vi "DAQ AO one shot ch 1.vi"(0 "device name":tag="Dev1", 1 "timeout (s)":dbl=1.0 format="%0.2f", 2 "stop (T)":bool=TRUE, 7 "Heater Voltage":dbl, 11 "error in":errorcluster, 12 "physical channel":string[](array[string])=["ao1"], 13 "channel name":string[](array[string])=["Heater"]) -> (4 "device name out":tag="Dev1", 15 "error out":errorcluster)   [LabVIEW 2019]
doc: "DAQmx NI ELVIS \nAsynchronous AO one shot \nchannel 1\nbug heater\n\nbuilt using the DAQmx assistant\n\nPaul K Dixon\nP3600\nCSUSB Physics\n\nCreates, edits, and runs tasks using NI-DAQmx. Refer to the NI-DAQmx Readme for a complete listing of devices NI-DAQmx supports.\n\nWhen you place this Express VI on the block diagram, the DAQ Assistant launches to create a new task. After you create a task, you can double-click the DAQ Assistant Express VI to edit that task. For continuous measurement or generation, place a while loop around the DAQ Assistant Express VI."
uses:
  <vilib>/DAQmx/write.llb/DAQmx Write.vi
  <vilib>/DAQmx/write.llb/DAQmx Write (Analog 1D DBL NChan 1Samp).vi
  <vilib>/DAQmx/create/channels.llb/DAQmx Create Channel (AO-Voltage-Basic).vi
  <vilib>/DAQmx/miscellaneous.llb/DAQmx Fill In Error Info.vi
panel:
  # "DAQmx NI ELVIS \nAsynchronous AO one shot \nchannel 1\nbug heater"
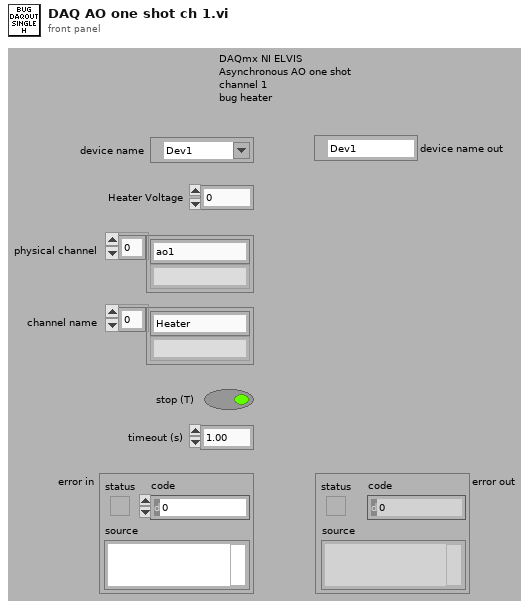
[diagram p1: front panel]
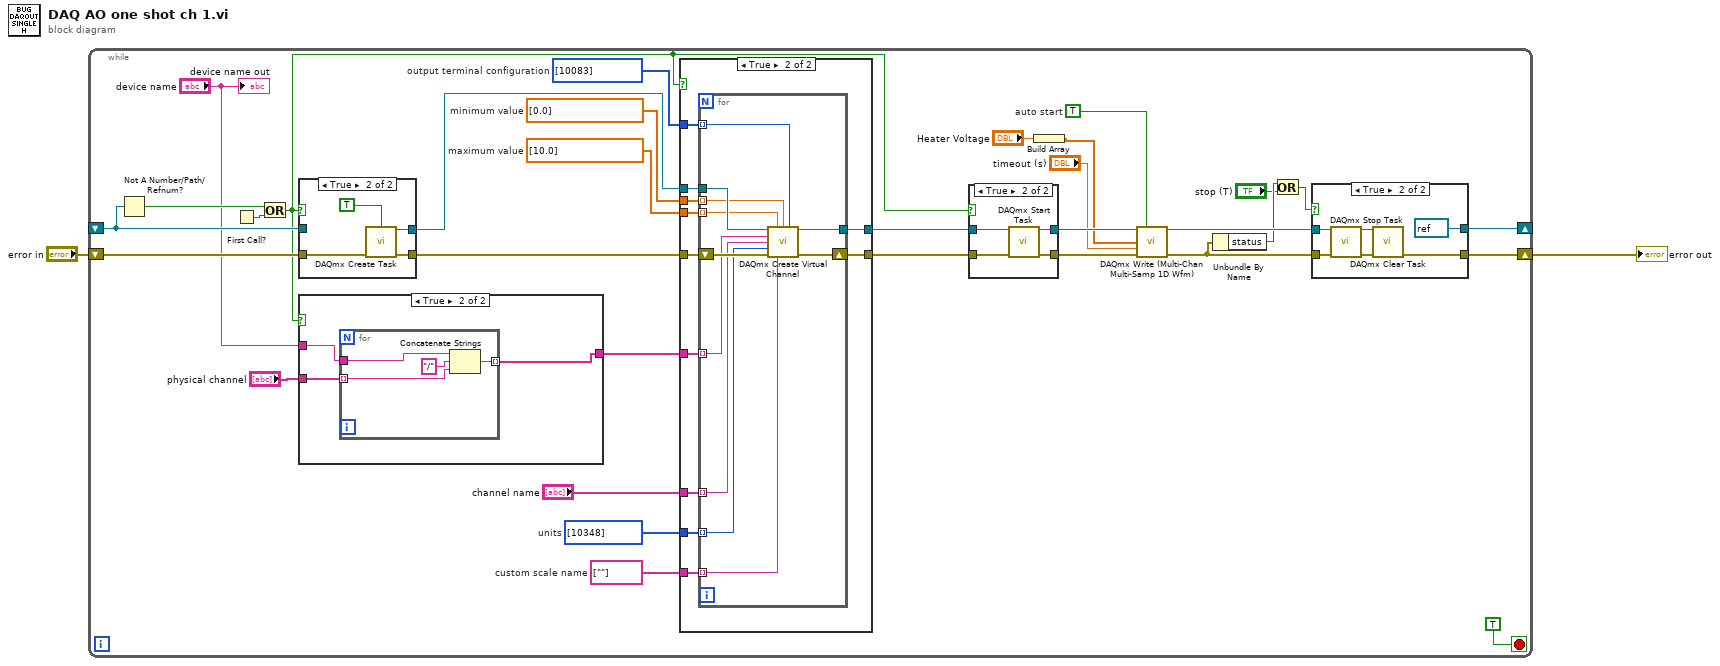
[diagram p0: block diagram]
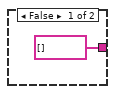
[diagram p5: hidden frame]
diagram:
  n1 = while {
    shift-right: [w11] -> _
    shift-left: _ -> [w31]
    shift-right: [w9] -> w1
    shift-left: "error in" -> [w32]
    stop <- TRUE stop-if-true
    w13 = TRUE  # auto start
    w19 = i32[] [10083] items=["Default"=-1, "RSE"=10083, "Differential"=10106, "Pseudodifferential"=12529]  # output terminal configuration
    w20 = string[] [""]  # custom scale name
    w21 = i32[] [10348] items=["Volts"=10348, "From Custom Scale"=10065]  # units
    w24 = dbl[] [10.0]  # maximum value
    w25 = dbl[] [0.0]  # minimum value
    n2 = Not A Number/Path/Refnum?(number/path/refnum=w31) -> (NaN/Path/Refnum?=w30:bool)
    n3 = First Call?() -> (First Call?: T/F=w33:bool)
    n4 = Or(x=w30, y=w33) -> (x .or. y?=w18:bool)
    n5 = case shown="True" w18 {
      tunnel: [w82 w86] -> w27
      tunnel: w31 -> [w82 _]
      tunnel: [w81 w85] -> w26
      tunnel: w32 -> [w81 w83]
      frame False {
      }
      frame True {
        n6 = call <vilib>:"DAQmx Create Task.vi"("auto cleanup"=TRUE, "error in"=w83) -> ("task out"=w86:refnum<k21>, "error out"=w85:errorcluster)  [unwired: 12 in]
      }
    }
    n7 = case shown="True" w18 {
      tunnel: [string[] [] w76] -> w23
      tunnel: "device name" -> [_ w75]
      tunnel: "physical channel" -> [_ w74]
      frame False {
      }
      frame True {
        n8 = for {
          tunnel: [w80] -> w76 mode=indexing
          tunnel: w75 -> [w79]
          tunnel: w74 -> [w77] mode=indexing
          n9 = Concatenate Strings(w79, "/" ("string"), w77) -> (w80:string)
        }
      }
    }
    n10 = case shown="True" w18 {
      tunnel: [w50 w59] -> w17
      tunnel: w27 -> [w50 w61]
      tunnel: [w49 w58] -> w16
      tunnel: w26 -> [w49 w60]
      tunnel: w25 -> [_ w57]
      tunnel: w24 -> [_ w56]
      tunnel: w23 -> [_ w55]
      tunnel: "channel name" -> [_ w54]
      tunnel: w21 -> [_ w53]
      tunnel: w20 -> [_ w52]
      tunnel: w19 -> [_ w51]
      frame False {
      }
      frame True {
        n11 = for {
          tunnel: w61 -> [w72]
          tunnel: [w70] -> w59
          tunnel: w57 -> [w68] mode=indexing
          tunnel: w56 -> [w67] mode=indexing
          tunnel: w55 -> [w66] mode=indexing
          tunnel: w54 -> [w65] mode=indexing
          tunnel: w53 -> [w64] mode=indexing
          tunnel: w52 -> [w63] mode=indexing
          shift-right: [w69] -> w58
          shift-left: w60 -> [w71]
          tunnel: w51 -> [w62] mode=indexing
          n12 = call-poly <vilib>:"DAQmx Create Virtual Channel.vi"("task in"=w72, "maximum value"=w67, "minimum value"=w68, "output terminal configuration"=w62, "physical channels"=w66, "name to assign"=w65, "units"=w64, "error in"=w71, "custom scale name"=w63) -> ("task out"=w70:refnum<k21>, "error out"=w69:errorcluster)  [unwired: 5 in]
        }
      }
    }
    n13 = case shown="True" w18 {
      tunnel: [w44 w47] -> w15
      tunnel: w17 -> [w44 w48]
      tunnel: [w43 w45] -> w14
      tunnel: w16 -> [w43 w46]
      frame False {
      }
      frame True {
        n14 = call <vilib>:"DAQmx Start Task.vi"("task/channels in"=w48, "error in"=w46) -> ("task out"=w47:refnum<k21>, "error out"=w45:errorcluster)  [unwired: 12 in]
      }
    }
    n15 = Build Array("Heater Voltage") -> (w3:dbl[])
    n16 = call-poly "DAQmx Write (Multi-Chan Multi-Samp 1D Wfm).vi"("task/channels in"=w15, "auto start"=w13, "data"=w3, "timeout"="timeout (s)", "error in"=w14) -> ("task out"=w10:refnum<k21>, "error out"=w8:errorcluster)  [unwired: 8 in, 1 out]
    n17 = Unbundle By Name(w8) -> ("status"=w7:bool)
    n18 = Or(x=w7, y="stop (T)") -> (x .or. y?=w5:bool)
    n19 = case shown="True" w5 {
      tunnel: [w36 refnum<k21> refnum ("task in")] -> w11
      tunnel: w10 -> [w36 w42]
      tunnel: [w35 w39] -> w9
      tunnel: w8 -> [w35 w41]
      frame False {
      }
      frame True {
        n20 = call <vilib>:"DAQmx Stop Task.vi"("task/channels in"=w42, "error in"=w41) -> ("task out"=w38:refnum<k21>, "error out"=w40:errorcluster)  [unwired: 12 in]
        n21 = call <vilib>:"DAQmx Clear Task.vi"("task in"=w38, "error in"=w40) -> ("error out"=w39:errorcluster)  [unwired: 13 in]
      }
    }
    "device name out" <- "device name"
  }
  "error out" <- w1
